vi "2020_day02.vi"() -> ()   [LabVIEW 2021]
panel:
  in  "Live/Test Data Src":bool
  out "Number of Valid Passwords (Task 2)":i16
  out "Number of Valid Passwords (Task 1)":i16
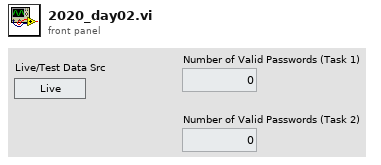
[diagram p1: front panel]
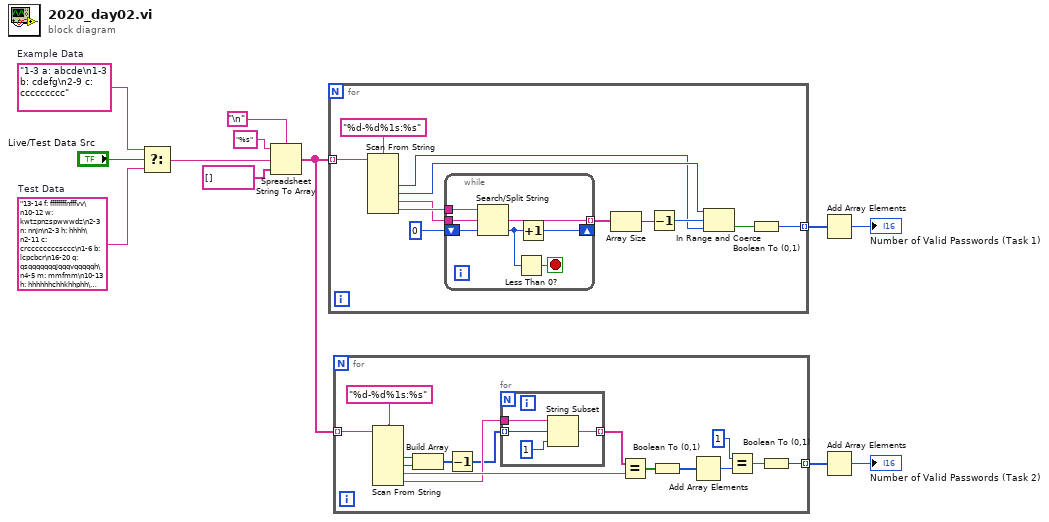
[diagram p0: block diagram]
diagram:
  w2 = "13-14 f: ffffffffnfffvv\n10-12 w: kwtzpnzspwwwdz\n2-3 n: nnjn\n2-3 h: hhhh\n2-11 c: crccccccccsccc\n1-6 b: lcpcbcr\n16-20 q: qsqqqqqqqjqqqvqqqqqh\n4-5 m: mmfmm\n10-13 h: hhhhhhchhkhhphh\n10-14 x: xxvxxxxxxvxxxwx\n2-7 v: tvvgvrvvv\n8-11 j: jjjjrjwljjzjkmc\n2-5 t: xtpftb\n4-6 m: mmmlmpm\n9-14 h: hhhhhhhhhhhhhchh\n10-11 x: xxxxxxxxxxx\n14-15 z: zzzzzzpzzzzzzzkz\n5-6 m: mwjmmw\n2-4 r: rrrr\n7-11 v: vvkwlmvkvkmbwvvvv\n16-17 j: jjjjjjjjjjjjjjjhj\n6-12 v: vjvvddtdpvvvldvqvdhv\n3-16 z: rktsvbkctznjkjzz\n5-6 r: hrrrrr\n1-3 d: ddxddd\n19-20 s: sssssjssssssssssssss\n17-20 b: bbbbbbbbbbbbbbbbbbbb\n2-4 m: mslm\n2-5 b: bbbbbl\n3-4 j: ljjj\n2-4 h: nlhbh\n4-5 z: zsmwfz\n4-5 j: jjzqj\n9-10 r: rrrrrrrrrj\n7-18 l: lljlgpmlltlzjltplln\n1-6 l: zbmljsljdszwl\n3-6 h: hhfhhqhhh\n10-14 d: vmddcdhsdzkxdddddddd\n6-7 s: psssssms\n1-10 j: cndjjjjjjjjjjj\n4-14 x: xxxdxxxxxxxxxxc\n6-7 f: fwfffsff\n2-11 v: dmmvlvsvvbbr\n7-8 l: dlcllllllll\n4-5 m: mmmmc\n4-10 m: zmmmlmnmrj\n5-6 s: ssshdsvbsk\n1-3 p: pppfps\n5-6 t: tttttt\n6-15 z: zzzzzzzzzzzzzzzzz\n7-12 m: bgshdmmkmmmmmfnmmm\n10-11 l: gclgllsllll\n3-4 d: dpdd\n2-9 n: kgngnrcxd\n8-10 n: knnsqnnnnrn\n8-18 f: qhwqbwnfppkffwhjjxf\n2-4 j: zwksc\n3-11 s: nkszjxwhcms\n8-11 b: tbbbbbbwbmbjk\n7-8 z: kvxfrzzzz\n2-5 g: hhwgv\n1-5 s: lmkxjbbsmnq\n2-7 p: spgxbpp\n2-8 z: xqzpztbvk\n4-7 r: wrtcfqrqcrlr\n2-4 g: gzgggg\n13-15 q: qqqqnrqqqbgqnqt\n7-12 h: dhxhbcqhhhhd\n7-8 l: llllflll\n5-6 d: ddbdfddwmndc\n3-10 j: jjjjjjcjjjj\n16-17 x: jhmqjpbpxsttjpcxrz\n7-14 j: jqjjjgjhjjmjjfjj\n5-7 l: zllllll\n9-13 d: dddddddxrdcsjdngbtd\n13-14 k: kdwkhqkkkkkknkk\n5-12 c: zcxwcbwfclccm\n14-16 x: xxfxxxhxxxxmdxxxxx\n10-11 x: xxxvxxxxxqxxxxxhx\n6-11 d: ddddddddddtddd\n1-3 j: bjbcj\n8-10 p: pppptppzpp\n3-7 z: zwldzgvztmbwwqwb\n4-5 h: hhhrm\n4-7 v: vvrvjvsz\n2-4 w: prsdkgxw\n1-4 q: fqqvqqqnm\n5-6 k: kzjbpkkkzzktkc\n12-15 s: ssvssssnsssdssgss\n3-10 w: wwfcwcwwwrjww\n6-7 t: thftndnvtztztb\n1-6 w: qgzppbcdjbpwmsj\n3-16 c: nccccfccrrcqhwcjck\n7-10 b: bfscxbdbnb\n4-14 x: xxrxsgxxwxptxxxdxdx\n1-4 c: jccb\n16-17 p: ppkppppppppppppwk\n2-10 z: wqtzzbhzkv\n9-10 b: bcbbqwcbbdvbzbfbsj\n6-11 s: ssssswsssssg\n3-7 c: wdcxzgtcrswqj\n4-10 c: xszcrmcsxccbwccxwv\n6-9 f: pffffffff\n7-8 k: wkhkhdkkkkkkrbkk\n3-4 q: cqqbqpg\n3-15 s: sswvssssswssssh\n19-20 k: kkkkkkkkkkkkkkdkkkkx\n11-14 d: dddddddddddddnd\n3-4 l: llll\n3-4 t: bvtvtrr\n13-16 b: bbbbbbbbbbbbbbbb\n16-20 b: bbbbbbbbbbbbbbbkbbbw\n10-11 v: vhvvvvvvvnvv\n1-6 v: xsvmvvxvkvv\n4-7 t: vttltqg\n16-20 b: bbbbgsjbxkbbbbbbrbqb\n15-17 c: ccccccchcccccxphcc\n1-3 w: cmwbtnzwwlhr\n2-16 j: njmqdfdsmrsptrjz\n12-13 r: rrrrcrrrrrrdhr\n11-14 j: jgjjjjjjjjtpjh\n4-5 w: wwstw\n5-6 w: mwrgwwmdwhzk\n4-7 b: bbdlbbbbc\n1-16 b: xbbhfbhbbbdbbdbbbbb\n11-14 h: hhjhjhhhhhhzhh\n2-3 t: jrtrt\n5-6 w: pdwwww\n5-16 m: mmhrmsvmxmvjdltm\n15-17 b: rbdbbbbtbfbbxbbbbbbb\n4-6 t: lzjtttqdpthkzrt\n3-4 x: xcxxxxxxxxxx\n15-16 z: zzzzzzzzzzzkzrcljz\n15-20 b: bbbbbpbbmbbbbbbbbbbb\n15-17 z: zzzzzzzzzzzzzcqnzzr\n3-13 t: tntttttttttttt\n6-10 s: jssmqsslsssddtg\n9-10 p: ppppppppjp\n9-14 d: sdxnfmpzlgvdcs\n5-6 c: cccscvcc\n2-4 r: rrrr\n11-14 v: vvcvvmvvvpvvvjv\n2-6 h: znfjphzqzdczp\n5-12 j: msdjjbjbgjjjbl\n4-7 h: hhhthkhhh\n5-6 q: qqqqqc\n18-20 q: pttqsnjcfchtfnqbjlqf\n11-12 x: xxxxxxxxxxxq\n5-6 j: xqbwjjcxjjljgj\n7-14 g: pdkdbzgzjvdvwggpnnt\n2-17 j: zhklmfrwspkgqbxjjdp\n5-17 b: bbbnbkbbbgbbxvzxhb\n6-8 b: bwhbbbbb\n6-16 q: lgxlqsqqwwmqrqqfgp\n16-20 j: jjjkjjjjjvjjjjjjwjjb\n1-2 g: vggg\n3-7 v: fvsvvxfvvv\n5-8 q: vdqqqqqqcrqqxq\n11-16 w: wwwwwwwwwwbwwwwnwww\n5-7 s: swwzsss\n3-6 d: hqwqcvdnqvh\n2-7 h: hsqhthghhhh\n4-9 d: dddtddddddd\n8-9 d: ddddddddd\n2-4 q: qqqsq\n4-6 t: ttnlqt\n4-6 s: sssszscs\n2-7 l: ssfllslplqll\n1-3 m: vmmlm\n6-13 q: qtqqqrqqqqqqqqqq\n2-10 d: zbldzlzssd\n4-5 n: nnndq\n8-18 b: wbbdgkvgscbdgqvxdj\n5-6 r: srrtrrrrr\n6-8 m: mmmmwbpm\n11-14 h: hhhhhhhthhhhhm\n2-4 p: pvpxpp\n5-6 g: ggvgng\n4-5 x: xxxtp\n3-10 v: vbvvzvhvvvvmvbcvvwrv\n11-13 d: ddddddddddxdldd\n4-5 g: gggggggggggngfggg\n7-8 j: jpjjjjhw\n2-6 m: jmfrmmhhsgbmmm\n6-10 v: vrvvvbvvvsv\n8-15 c: cctrcccpccccgcc\n14-16 d: ddddxdsdzwdddwdsddh\n5-6 m: mmnmmb\n2-6 d: dtwlswdnlkn\n12-13 x: vldxvmxcnndzx\n4-6 k: kkkxkm\n1-4 p: pppp\n11-16 b: bbbbbbbbbhdbxpbbbpb\n1-5 j: jjjjjj\n6-8 q: zqwdqszvqwqbrmhfqqm\n2-5 q: nqqczhb\n12-17 v: vvvvvvvvvvvtvvvvpv\n1-3 w: wwlww\n9-11 n: nbndcjnzntnvjnk\n3-4 q: qqcr\n15-17 p: plppppppppbppppplpp\n1-2 c: cvdlsccrccldccvfcc\n4-5 p: bpppcp\n19-20 d: dddddddddsdddddddddd\n2-4 t: bwbtmjbgkdlpjkrxt\n2-5 l: llxdblrcvnpclt\n11-13 b: bpbbbbbmbbbpbtcbbbzm\n6-7 p: ppppppp\n5-18 m: mqmmqpmmmmmwmpmzchms\n3-6 g: ggggmggkgg\n11-18 z: wjwlzzptzzzwbmzzgz\n5-7 b: bbcxbfbwbbcn\n4-5 p: szppp\n2-12 b: bbbbbbbbbbbmbb\n6-10 m: jmmmmwmtmfcwwxm\n4-5 m: mrqzmmmptfkmch\n13-15 q: qqqqqqlqqqqqqqqd\n1-5 b: kbbbnb\n4-5 t: qdtttszwwppbtllp\n12-14 c: cccccccccccccm\n4-5 g: gggdhg\n1-4 b: wbtbb\n3-6 d: ddrdgbdvdv\n14-15 x: xxxxxxxgxxxxxvdx\n13-18 l: lllllllllllllllllll\n5-7 p: zjsxppv\n4-13 v: vvvpvvvvvvvvf\n17-19 q: qqqqqpcqpqqgqqqqqqmq\n1-5 r: rlmrrr\n8-9 j: jjjjjjjjw\n2-4 q: dswq\n16-17 z: zzzzzzzzzzzzzzzzzz\n4-7 h: hhhzhhw\n11-12 l: lllllhhpllllqlllln\n11-12 h: hhhhdhhhhhrhh\n3-4 j: pkthmjsjqx\n15-18 b: bbbbbgbbbbbbbbbbbh\n4-5 j: lsxklmdwmhj\n1-2 p: pptp\n8-10 g: fgggzrnggg\n3-7 k: njkdhpkpqtqxhqwkp\n10-11 l: llllllllllz\n12-14 q: qjqhkqmqqwqgqcg\n1-3 m: mmmm\n8-19 c: dwzvhvbcpdbhcnrlcncx\n3-7 x: xtxjljw\n6-18 t: pttgnchttttttttqtt\n3-4 p: pppxpp\n15-16 k: kkkkkkkkkkkkkkvr\n2-3 x: dxxmx\n12-20 m: mmmmmjmmcmdmmmmmcmmm\n6-13 h: sthvjhlhfhxlhb\n4-5 t: pbrlttgmmwztxtrt\n3-7 p: dpptmppp\n7-9 p: hpppppppp\n3-4 q: qdgqqq\n1-4 c: cffcrkpdczhbj\n1-8 d: cqdwddlrddd\n9-10 n: gnkmnxnzmn\n3-4 k: kkxx\n1-7 d: vnddddn\n8-12 l: jllnlcllllllllvllb\n1-4 n: nnnnnhnnnn\n9-12 s: tssssszsssssbt\n8-13 h: nhnhdtkjbsfvbsh\n2-4 v: qmvs\n3-6 c: chcxccch\n1-5 d: ddddd\n11-15 l: pklllvllwlmlcklllll\n1-3 v: dvkbwsgjzqzzjmznd\n5-6 j: zjjjjjs\n1-4 f: vbffrwfr\n3-5 x: xxxxxrfdxmnbkrjbdzcx\n16-19 s: spsssbmrpbwrhqssgft\n13-15 v: vvvrvvvvbvvvvvv\n6-9 q: lqfqgcwtdqzgrqqp\n3-5 w: fwpwx\n7-8 h: hnhschhfphjzphwh\n2-6 r: rrrrrrr\n8-10 h: hhrhzhhttm\n9-16 w: wwwwwwwwfwwwwwwh\n2-3 n: zbnfnlpcnjqftpv\n14-17 k: rqwlkzqczczrlktcl\n6-7 f: ffffffff\n3-6 k: nndkjtpjzpmkkr\n12-17 p: gpppbpmjpptpfnzpb\n16-17 n: nnnpnnlnnnnnnmnnnnnn\n4-6 r: rrsrwr\n4-7 x: cnljrzcj\n7-8 s: srgtqlmc\n8-10 n: nnnnnnnvnn\n2-5 g: ggqggb\n7-8 h: hhqhgpxb\n4-12 b: bxbchbbbbbbbb\n2-4 z: qfzng\n6-13 m: pcmmwdkmzlstn\n3-4 v: qvdc\n2-10 t: tktttttttmt\n9-15 t: tttttttttttpttw\n8-13 p: pppjpppkppdlv\n6-9 g: gggggngqg\n2-9 k: lzvkqkkkkk\n8-12 h: ldpnjvchhshx\n5-14 c: cccccvrccccdbccchjc\n14-19 k: kkjksgrrkklhkkkkkkt\n5-15 r: hrrrrrwmrlrgrlz\n7-17 g: hbjtgsxbgrgggcjlk\n4-6 q: lqcbqvzqrqzqxqnqd\n5-8 x: xkdxsxxf\n12-16 m: vxlfjgzgqhxmlvmmqmm\n2-13 c: vccvjvqrgrsrqv\n4-6 l: ltlrlpvnl\n12-16 p: ppptdppppppcfppzpgsm\n18-19 q: qfqpvwpwjqvlnrmvsqq\n5-6 m: mmmmmh\n6-7 m: mmmmsls\n3-4 p: pvcg\n6-7 h: hhhhhhj\n1-4 g: gkggc\n3-10 n: sqsndtgnjbnljnn\n5-11 h: tcmlhlnbfnhgt\n9-10 t: ttttttttxl\n6-8 x: mxvxxxxhxxccbx\n9-16 g: rgggthgxggdggjgg\n7-20 w: wwnwwhvmtwnvwwpzdxvt\n13-14 t: tttmttlttgttlptt\n5-6 f: ffffpg\n5-7 z: qzzzzzqzz\n1-3 b: bfbfdhkwdzttcldtr\n5-8 n: nnnnrnnqnnnn\n7-18 m: hgnrbdmvmzqmhnhhpww\n2-6 h: rjghpwxhn\n5-10 m: bjqjmmnbvmlxpvvdds\n3-4 v: hvjttv\n4-8 n: nnpnnnnnn\n1-10 g: gzxghcgkggggtxg\n4-6 b: pbgblbbb\n4-7 c: ccccccmc\n2-4 g: ggwgtzvxqhjqphfg\n3-5 t: htdtt\n8-9 t: tttttptttttt\n4-5 v: dvvvd\n6-12 p: skzhnpblmpppcptfpll\n15-16 l: llllllllllllllvp\n6-11 b: mbbbbjxbbmbbf\n2-4 t: mtqwtnt\n2-4 h: wfhkh\n5-6 w: wwwlwwwkw\n7-8 k: kskkkktz\n5-6 g: rggqcv\n2-4 z: krmw\n2-4 q: qqwqlrqcbxlxbpqg\n14-18 m: mmzmmmmnmmmmmtmmmm\n1-5 p: pqwfpnp\n3-7 w: dwwxdwgwwksm\n8-11 g: bkmcfcddjvw\n7-9 s: srsszspss\n3-4 r: rjrsz\n12-14 k: kkkkkkkkkkkgkl\n13-14 f: fffffffffffffh\n7-9 r: qgxpglrlr\n4-6 l: xflkll\n2-9 d: gdddddddrqdddd\n2-3 k: zskkzq\n3-4 z: jzrtwgmtl\n3-4 b: bnnbbx\n1-9 r: rhmrwwrfmsb\n7-10 b: btbbbbbbjbbb\n7-8 t: lmttpttq\n1-4 s: rcls\n11-12 k: kkkkklkkkskq\n14-15 p: ppppppppppppppp\n3-7 l: dcslvkjgjcdk\n1-6 l: hllhllpl\n6-9 z: zdlqztzzkzz\n10-11 r: rrfrrrrrrrqjpkkrmrrh\n4-5 v: bvpqvvkvrxnvzmghbhmx\n10-11 v: vvvvvjvvfcvvcvpj\n10-11 j: jjjsfhdmjtcvbzj\n4-5 z: zzzzzz\n14-15 l: lllllllllzlllkcnl\n3-8 c: dchcjjrccvm\n12-14 b: vrwbfbqbbbbkbhgqjjh\n8-9 g: stggqgctgpgggctt\n15-17 p: pppppppppppkppqpp\n7-8 q: qqqjvqhmqq\n3-4 x: xxxxx\n7-8 g: ffbgglgzpjgqvnglpsgh\n14-16 r: rrdrrrrrrrrrrgrrrd\n10-13 l: lllllllllllll\n6-14 q: qfqzqnqqmhqqsp\n2-3 q: qqqqq\n17-18 f: ffffffqfffffffffftf\n11-13 h: hhhhhhhhhhmhz\n3-10 c: cccmcccccfzc\n8-12 v: vvvvvvvvvvvvrfwrvv\n3-4 v: vrnx\n1-12 v: gfvsvkvvvzvcvsv\n9-10 b: lbtgbbpcfbgb\n6-8 f: fgnffkfshhfbfc\n8-10 w: wwwwwwwwgpltzwzk\n7-12 b: btbbjbhbbpbbqsbbbvp\n11-12 r: vfcvrrrzrhvc\n19-20 g: gggggggggggggbggggjh\n11-14 s: sfsvsfsswsssscxssm\n4-6 c: lcclcc\n7-8 g: gggggggr\n10-14 g: gdcpmgxlgggggtgbgg\n2-3 b: bktb\n9-13 k: krkkkgkkkkvkkk\n2-12 f: bwtgngzflzcfchx\n2-4 m: mmmmmmm\n10-12 b: bbbbbbbxbbblcbpb\n3-4 c: ccct\n6-8 r: kgqvrrrjn\n10-12 f: ffffffwfffff\n6-7 c: ckcjcjccc\n10-12 l: lllltllllllxll\n3-6 q: qqgqqlxqqq\n4-5 b: nbbbbb\n7-11 r: rrrrrrrrrrrrrrr\n10-11 s: sssssssssss\n1-6 w: wwwwwwwlww\n5-7 l: lrlmlll\n8-12 c: fbcmjxccqcwc\n9-10 b: ljmbxwbbbbbhbbb\n2-4 h: shwgvlw\n15-17 t: ttptttttktttkttttt\n2-5 d: dddgdd\n2-14 x: xbbtnzdvbszrlxl\n8-10 c: cccccccbcx\n10-12 k: kkkkkkkkmkkc\n7-17 r: rzbcshqhmrzrktzdr\n5-16 k: kvkkdkkkkkkkkkklk\n1-7 p: hkplfbjdhsh\n1-6 z: pnzzzz\n12-18 m: mmmjmxmmmmmmmmmmcd\n5-7 k: kskkdbsk\n9-10 b: bbbbgbbbbw\n4-6 c: cccccjs\n19-20 w: wwwwwwwwwwwwwwwwwwwf\n7-11 j: drzjhxkjjjkwr\n10-15 c: cccfckccccdccxc\n1-3 d: ddddc\n13-14 j: jbjjknjjjjjjjjjjjzzc\n1-4 m: mzmftx\n1-4 t: rttt\n12-17 t: tltqttzttttjwcttrwtt\n6-10 m: rmfmrnmmmdmqp\n6-15 p: jpfpppwppppppznpppp\n4-8 p: mppxctpb\n2-4 z: gwzzrn\n3-4 p: ppfpp\n3-4 b: bbbh\n11-17 l: llllllllllllllllhll\n4-6 m: mmmmmmm\n4-6 c: ccccjx\n11-14 g: gggggggggggggg\n3-4 l: llflq\n9-13 p: pspvvcpkpcpzpfpk\n1-4 n: nhwn\n6-10 j: jjjjjjjjmjj\n9-12 p: ppgpwxpplgppzpppwpp\n10-14 h: hhhhhhfhhhhhmxh\n8-10 l: llllllmcwfl\n7-8 h: hhjhhhps\n8-11 v: grvvvgbvxvvlhvvbdvr\n5-6 m: fmjjbmp\n1-2 x: xxhd\n11-15 n: nnnnnnnnnncnnnm\n1-8 g: jgggbggd\n13-15 l: lshllllllllllll\n5-12 r: crrsrrrrprtrr\n10-16 k: hkkkkkkjkgtkkkkkq\n5-16 j: prxjxjjdxzjjvjjwfj\n7-8 k: pdkkkkkzkzw\n3-4 s: sstg\n1-5 x: vxxxb\n10-16 s: tqmzsfksjzfmlqzsdb\n2-5 r: rcrxjr\n10-15 v: jcbvvvhvvvkwrgvvvvv\n4-6 n: nnxnnpnn\n13-18 l: llllllllllllbllllgl\n9-11 g: vwqgnrzlclgqtp\n2-3 f: fpms\n3-5 l: llllllll\n7-12 x: xcvxzxxhxxxxxxxxqxxv\n6-10 b: fcfpwbmbhbpbbqkkbxb\n8-11 z: nrnzzqzzzzck\n8-9 g: nggdfgdgggfggg\n2-6 d: sdztkkfvpkddggdxd\n10-14 g: nhdstmlfxcggcs\n10-11 g: ggzfglgggmcxgjh\n3-13 x: cxjxxxxxxgxvj\n9-10 h: smlxphtmkhf\n7-8 v: rhdvgcvrdvvvvvxwvssh\n7-14 n: nnnnnnncnnnvnn\n3-6 z: zzzgznzz\n6-10 l: llwmgllljllll\n4-5 v: vwvvpvw\n7-8 m: mmmmqvmqmv\n13-14 z: zzzzzzzzzzhzrcz\n3-8 h: bdmhcxpgbpjvwfmh\n3-5 h: nhhjk\n11-19 b: zrrmrqbfvwbnmvkvbzbv\n3-8 c: ztwqhccmwzvcbxjjrc\n4-9 h: hhhhhhhhh\n2-15 d: lddzlxhkscrmfbd\n3-9 s: kpscwnwzj\n10-11 w: zwwlwxwwwwwwww\n4-5 v: dpvjr\n1-3 d: ddtd\n3-6 x: xxdfxxxrbdh\n3-6 g: dghwgxg\n8-10 z: zzzzzzzpzz\n13-15 p: pjpxpppppdcpphlppjp\n6-16 j: jjjjjljnjjjjjqjjjwx\n11-17 f: fffffffffflfpfffxff\n8-10 j: jjjjjjlwjkjrdjjjj\n8-9 w: wwwwfwwdkww\n4-9 x: qpxbhxwxxkx\n5-7 w: wwwwbwl\n1-6 m: mmfrmmmm\n8-9 l: lllllvlsl\n3-4 d: dddd\n6-8 c: cqcptcfcgcrzbjcccp\n10-11 k: dccpkmkkgkkdzkkkkkk\n3-4 j: jjjr\n3-9 h: hzhwhchzhjg\n7-8 g: bxgnvvzfsbggdgg\n2-17 f: ffffffffffffffffffff\n7-13 g: ljggdgztggvgtggg\n9-13 x: rxlxrxxnwqxpcdxq\n10-11 j: jjctjjjjjfjj\n8-16 k: zpzskgkkkvsbxhsk\n4-5 l: llljl\n2-6 b: bbbbbb\n1-3 w: swww\n6-8 r: rrrrrbrbrr\n8-9 t: tttttttth\n3-5 s: sssss\n3-14 q: qqxqqqqbblqqcqmqsq\n7-8 v: dmfvccvvvbvmwjvvvqfv\n5-7 v: qvvvvvvvv\n4-9 c: cgcgvncctwrtv\n3-5 p: ppnpppp\n13-15 h: hhhhhhhhhhhhhhhhnhhh\n5-8 r: rrrvpgrdbhrc\n2-9 q: szlqwzwhqxbxkr\n5-6 c: cwrmhxcpxchzccb\n4-6 z: zzjczz\n12-14 p: pwqkbphzplxhnpm\n8-13 t: tkkzjttrstbtwttd\n15-16 m: mmpqmxbxdzmqmmmb\n4-6 c: ctcpczdd\n2-3 j: fdjjj\n15-19 k: kkkkkkkkkkkkkkpkkkwk\n2-3 c: cccc\n1-2 w: wwfqwwgpmv\n2-3 h: wfzmhm\n3-10 s: wbsbvhfxjgxfqstwqn\n15-16 r: sxrzvkqpqmgzgtrr\n3-5 m: fmmtmqjxzss\n12-13 k: ddsnpkfvknhwq\n5-11 z: lzwvzhtzzzz\n12-13 t: tttttttttbdgtft\n14-19 g: gggggggggggggggglgnv\n3-4 r: rrrr\n3-7 h: xchhnhh\n10-11 n: ndnjnnhnnnk\n5-7 l: llllhll\n3-5 p: ppppb\n11-12 s: rrsjzvswsdtxssv\n2-10 z: ztxzzzzzztzp\n16-17 m: mmmpmmmmmmmmmmmmmmq\n1-6 b: wkbfntzw\n10-14 n: nnnngrnnnnnnnnnn\n1-3 b: pbdfsbbp\n6-13 n: brnwnhnnsnnrwncnmz\n2-11 f: mlhpdjflklzmhxt\n1-2 f: shzsffl\n8-16 k: kkkkkfkxfwnslkkm\n13-14 b: bbbbbbbbbbkbqbb\n2-7 x: zdxxxxxx\n6-10 h: hhthmpvhnlk\n6-7 p: tppfpqpcppppxpmpcpp\n3-5 m: grmkm\n5-11 w: vcwbwwwbwwswnrdwfwx\n1-6 s: sssrssssx\n13-14 j: jjjjjjjjjjjjgj\n14-19 q: sbqqzqnqnlzdrlqqqtkl\n3-4 t: btdttvzrvnjst\n1-7 s: ssbsssmhssssdsc\n3-4 z: vcdzj\n6-13 v: vvvvvvvvvvvvvv\n2-7 t: ttttgpthqhmth\n5-9 z: zzzzwzzzl\n10-15 w: wwwwckbzwwwwkwwlrwb\n2-7 r: wjrbdzrjxrstrc\n1-8 z: dpzzzvcsx\n4-6 c: nccxccvcccczcccdc\n1-10 c: cccccccccc\n3-7 d: zdmdpdntdpzncdbff\n5-9 x: xvlvxldrxxmbdcdxxxz\n6-7 p: ppplppjcwcpp\n2-7 d: pwnhpdd\n2-3 q: hqqsdqxs\n6-9 t: smttzjmktq\n7-9 t: ttttttttp\n4-19 w: wwwrwwwwwwwkwwwwwwnw\n17-20 s: cssvssssssssssssssss\n10-11 s: srssssssssss\n5-6 f: ffcfjt\n3-4 d: ddgdddddddd\n2-15 s: sssssssssssstsssssss\n2-4 c: kmccnnt\n2-3 f: ffff\n10-14 s: vspjssnsssssshvsq\n9-10 k: skkkkkkfxkkwk\n3-5 g: mgnggjpgspcf\n4-15 z: zzzdzzzzzzzzzzzz\n3-4 c: cgcc\n6-7 s: sssssjs\n2-4 z: ztzz\n17-18 w: wbqwwnwwwmwvwwhgdnl\n13-15 d: dwddddddddddwdddd\n4-7 g: gzghgcnq\n3-9 n: snnnnnmll\n2-7 j: sjhtsxj\n2-6 h: khvzdhhr\n2-10 t: tttttttttttttttt\n4-6 x: xxglxwjrx\n3-4 r: rjrc\n5-13 b: bbbbbbbdbbbbbb\n3-4 q: qqrhqq\n8-12 g: ggggkggdgggbg\n3-12 j: jjjjjjjjjjjjjj\n1-5 c: cbcch\n10-11 r: rrnrvrrrrzn\n4-16 j: jjjpjjjjhjjjjjrjjjv\n8-9 f: fffffzdsvfccfr\n14-16 f: ffzfjfftfffffffffff\n2-8 n: ngnnnnntnnnnr\n6-11 n: nchnnvnnnndn\n4-5 w: sfwvm\n6-14 s: ssssssvsspssqhsss\n3-4 m: sjjb\n2-4 d: dnkjd\n3-9 s: twsgkmqstq\n6-14 f: ffffffffffhfff\n10-15 w: wmwlwwwwfgwwjrzwwwww\n3-11 f: fffffkxfffffmfff\n1-2 l: jlrpl\n3-14 p: pbnpkbppxhppmpp\n1-14 v: bvvvtvvvvbvvvh\n3-4 s: zssvs\n3-4 l: llljrlk\n8-12 f: ffcfffczlffff\n3-13 m: xsmgpvzsrrwmxtbktsrj\n5-7 j: qxvjjlqjjjjj\n3-4 r: rbdwg\n13-14 d: dddddddddddddg\n10-12 f: lqvhjnkfrfffv\n6-7 n: njnnnhz\n11-13 v: vvvvvvvvvvvvs\n12-13 v: nvvsfvvvvvnvdvjxvvv\n2-19 s: slsssssbsskspssssts\n9-11 n: nnnnnnnnnnm\n4-5 j: mhngjjrhjcjkjw\n12-18 p: pnfwppppprsqrppltppp\n9-13 s: wsssfsjsssfssss\n6-8 b: bbbbbzbj\n9-12 c: lcccccrccctv\n7-11 w: wbdwwqwwkbwws\n6-19 c: cccrmldccfhtvclcccc\n9-14 h: bhhhhdhjkhhhhm\n7-15 g: gkgggggvcgggghgggz\n4-8 k: kknklwkkkg\n10-13 c: ccccccxcccccccc\n10-14 c: ccbcfcccptcczbcc\n8-9 s: scsssssss\n1-7 v: bvvvvvvvk\n4-8 s: dspsskkstklsz\n9-10 b: blbkkzbvvpbhbbbb\n1-2 m: qgntnbccqm\n7-14 w: wwwwlftgspwmwr\n4-13 n: tnxmnnwwnnlnnnnz\n3-5 c: cwzbs\n3-6 d: dddddl\n6-8 s: qsfssrnsst\n1-2 l: llxcx\n9-11 g: zhzkcbglvgw\n5-11 f: lfzgtbcmzzw\n6-19 m: gcbgjbqrdkswqhmxjct\n1-3 z: dzzz\n9-13 t: wttftcddttmtttgttnvt\n14-15 z: zzzzgtzzwzzzzzzzzz\n1-11 q: qqqqqqqqqqqq\n4-5 j: rxjjjxjwjjj\n3-5 v: gqjhjvlvlbmkgssd\n16-17 q: qgcbftwncjhdzwqmw\n1-3 g: tjftgp\n11-16 l: rlllllllllgglllm\n4-6 z: zprzvrfbpblf\n7-11 j: jjjjjjjjhpjmjj\n3-4 l: ltlrblllwljljlc\n8-11 k: kkvkkkkkbqkskrkkd\n5-10 r: hjrcrrrdvtrkrvrxrr\n5-6 x: xxxxpx\n13-16 g: gmggggggcggpwgghgt\n3-4 h: hzzp\n13-15 h: hhwhhghhhhhhhhh\n3-5 t: mlftttt\n8-13 c: cccccvcdccccfcccccc\n1-6 k: kczzpq\n8-14 t: rtcttttgtttttgtttz\n6-7 l: lhsvlll\n1-2 x: cxlr\n8-10 t: rtbtttttsblttttb\n11-14 z: zzzzzzzzzzdzzzz\n2-3 t: ltttbthjdxwbxrv\n5-6 x: xxxxxxxkx\n8-12 f: fffffpffwfng\n5-6 x: xxxxflxxxxx\n5-7 d: ddddvvk\n4-8 j: ttjjjjhj\n2-5 p: rtrmpksjdvpplmrkl\n9-11 s: ssshsskssssssr\n5-8 j: wjnjjvjjfjjhf\n4-6 q: qlpcjqqqq\n13-14 m: zctdnmkjstxbmmfqtns\n4-11 n: nqntnngnvmnknrnwnnl\n3-5 d: ddfvdnkd\n9-14 j: wsznlrpljmjwjjjkmtk\n2-6 w: wlwwwww\n9-12 j: jjzjxjjjjhjp\n10-13 v: zvvvvvvvvfvwlvvvv\n3-18 x: dzxcqgwxpwxvpmcxxdxx\n2-3 w: wsgwwd\n3-20 n: nrnfxnnnnlnnnnnfnrhp\n3-8 f: fmvjwsffvxjfnlw\n5-6 l: llllcs\n3-5 b: bbbbbbc\n2-7 l: rlwkflnsm\n4-18 m: dqskhdqgmrpbgtmdnp\n4-6 r: grpxzr\n5-7 m: mmmmmmjmm\n7-8 b: bbkkbbkbb\n1-4 r: rwrtr\n5-6 g: gggcggg\n4-6 l: qlcbwrsf\n16-18 t: tttmtttltvtttttxtrtt\n3-4 z: zzzz\n6-10 g: gggggtgggg\n12-15 f: tffffffffqrffvvftffh\n10-16 w: wwgwwpwhqdwhwpbw\n5-7 m: mpmmmmm\n3-5 b: bbxtbbb\n5-10 x: xxxxbxxxkjkx\n10-12 b: bjbldbbbwbxg\n3-4 g: gnggqgg\n2-4 s: sstst\n6-10 j: jjjjfvjjjj\n16-20 r: rrrrrrrrrrrrrrrrrrrr\n4-12 b: bbbxbbbbbbbbbbbbb\n3-4 k: kkpk\n4-7 s: ssssqsh\n10-13 b: vbzbbbbnblbbb\n12-14 f: rgqffrfsvftwff\n2-4 x: bfxvhmsxnqxz\n10-12 c: ccccccccccbcc\n1-4 l: llxbmjpll\n9-14 f: ffhfmpfffffzfgcg\n3-4 n: ndfm\n1-6 k: lkmdzgfbkfktkkvkw\n12-13 q: qtkqqgqbqtqgvqqqzq\n7-9 d: ddddddhddsd\n4-11 j: kdqjjjjjjxg\n4-6 k: kkkgkm\n6-12 n: nnnnndtnnnnnnv\n2-6 c: dccccdc\n10-11 v: vvvlvvvvvvb\n7-10 w: wwwwwcwtzwkpvjqwsb\n1-5 x: xxxxxxx\n5-8 g: dhggzggsggggglgggg\n8-9 t: dttttttdtfnt\n11-17 g: cqgglgtwgggcbwjvwg\n1-2 t: ttttt\n16-17 j: jjjjjjjjjjjjjjjjjj\n4-7 k: lkdkhkkkfk\n15-17 z: zzzzszzzzzzzzzwzlz\n3-13 w: wwswwwwwwwwwfwww\n5-12 h: mstzhsghhhhnzmdrh\n10-12 h: hhhhhhfhhphhbhhk\n3-4 j: jjsd\n11-12 k: kkkkkkmkkmfd\n19-20 d: ddddhdddddddddddddxj\n7-8 g: gggjggrg\n4-5 m: mdzmv\n3-4 w: wwww\n7-8 b: bdbwbbbbb\n2-12 q: dxqqqqqjqqqlqq\n3-6 w: wwwwxwh\n9-11 s: smhnkssssssstxj\n5-6 n: nnpnkj\n7-8 s: qsgdxkjs\n9-14 m: mmmmmmmmsmmmmv\n1-3 v: vvcvv\n2-5 x: kzxgjttwxspclfx\n5-8 c: ccctpcckz\n5-6 h: hhhchthqxchh\n3-7 t: hnrcqdtttmtxtnmhcf\n2-4 v: vvlz\n4-5 k: kbgkl\n9-12 x: mhzpjqtxqnfrcnwhk\n7-11 z: slztclzvxbzmz\n13-14 l: ldllllllllllkcl\n1-2 l: fslcthfv\n12-16 b: bxbkbbbbbbbbbbbb\n1-4 r: rrmr\n8-11 d: dddfdpdddtdd\n17-20 n: nnnsngnbnnnnnnnncnnn\n1-16 x: xxxxxxxxxxxxxxxxx\n2-4 z: zqzv\n1-4 m: fnwm\n2-3 j: jqvd\n10-12 h: ghhhhhjhhchg\n14-15 v: vvtvvvvvvvvvvvv\n4-6 f: ffffff\n8-20 g: tgghjfglrzggggcxhcgg\n9-11 p: pvpmzppppkpk\n5-18 x: xxxxnxxxxxxxxxxxwlzx\n10-11 m: mgdmrfchqwmfmrlnq\n7-8 g: gggggzxs\n4-6 n: vjnchzknzbvnvn\n17-18 p: pppppppppppkppppjp\n6-8 d: dddddfddld\n1-4 r: brrr\n2-10 m: mzmmhqmmmmkmmwm\n8-15 f: cfjwxkgmfkxdmwxf\n3-8 c: djskjzcmwjcz\n2-3 k: hkckkjbztrggrffvxwm\n11-13 d: krddnddddrddgdddd\n4-5 f: zjsndf\n4-5 r: rrrgl\n1-2 z: tsbn\n1-11 s: sssdwtjssssskkszms\n6-16 x: xfxxtxxxxxxdxzxmxx\n5-13 m: mmmmmmmmmmmmmvm\n2-4 z: zdzj\n3-4 d: dddd\n3-4 n: nnmnkv\n14-16 d: dfddddddddddtddddqdd\n5-7 n: jnnnnnnj\n8-16 q: qqltjqqqqqqqsqqfq\n10-14 s: sssxsmsssvqjssss\n6-7 w: wwwwjwwxwd\n2-5 m: mzqcndqmnmmgwmsspm\n9-10 k: tkkkkrkkkhkk\n3-5 r: rxrrrrr\n7-11 c: glfcdqrcnfhc\n8-9 r: rrrrrrrjd\n7-8 d: ddddddlk\n2-7 j: pjsmjjr\n2-4 x: txxx\n13-15 f: ddkhqfnbcmtwvbf\n7-11 n: nnnnnnnnnnvn\n7-9 m: jmmmlgmmthlrm\n8-13 w: wwwwkwwgwwwwfrwww\n2-6 d: drdrhn\n8-10 k: lnkfrvgkzkchq\n4-7 z: lxjzzzzhzprrzzzpcwj\n1-2 s: lssc\n2-3 n: jmkcngpn\n3-9 x: xxmzxnxxxx\n3-12 v: nqwshwqgfnwvwvnf\n5-8 m: zmmmmmmmqlkprv\n1-5 q: qpqrqwqsvpjqf\n14-18 q: qqqqqqqtqqqcqqqqqq\n13-16 v: vvvvhvvvvvvvrvxdv\n2-6 r: rrlrrrk\n6-8 r: hmsrxsrkprdrrrl\n14-16 s: sssssslssgswssssss\n3-11 t: ctttvsnfcstzktktb\n1-11 c: gwfbddphwnqcmf\n3-18 h: hhhhhhwhhhhhhhhhhs\n7-9 c: cjjcrtpvctccfcc\n6-14 f: fffffgfffffffff\n8-15 z: zzzzzzzzzzzzzzdz\n9-16 d: ddddbdddhddddqpd\n1-2 q: qffc\n3-5 l: grcsjln\n12-13 q: qqqqqqqqqqqqq\n4-5 q: qqqlk\n1-3 w: wwwx\n3-4 w: kwwf\n5-15 m: pkwmgmmxspzxhmmrmp\n5-18 t: ttfthsbwntpcnttmwtc\n14-15 p: pjpjwppkpxpqkpf\n1-3 n: nnnn\n8-9 j: jjjjjjjbxj\n4-6 w: gfhwfwwmfx\n8-11 k: kkckkkknkkkk\n13-14 m: mmmmmmmmmmmmsqmmm\n2-4 s: tsrz\n9-13 j: tjvjqpnjjjlkwjjljrj\n3-4 f: xwfgf\n2-7 h: rhxshbh\n10-18 j: jjjjjjgbjjjjjjjjjjj\n5-14 n: fnwnnnsnnnncnpnn\n9-13 h: qhhlnhhhqhhhm\n3-17 h: hhfgzkhhjhrbhwdcpbnh\n2-4 c: qccrblqtcd\n13-16 s: ssjssqssssqsxssw\n10-15 n: nnnnnnnnnqnnnnf\n2-3 m: nmtl\n2-4 w: wqwdt\n4-7 v: vvvvvvvvvvv\n5-6 w: wbctwwwgj\n4-6 q: qqqttqzzwsxp\n2-7 r: rcrrrrrr\n10-12 d: sdmddcfdddzvdddddq\n1-15 f: ffffffffffffffffff\n3-7 r: rrwddcjgr\n2-11 t: tttttgttttttt\n3-6 n: nhxgnqnnfs\n1-3 t: pqtwt\n8-17 r: rrrrrrrrrrrrrrrrrrrr\n3-16 t: tktnpjtcthrhtqltq\n5-6 h: kcmkkqdrbhhxm\n3-4 l: llll\n1-14 g: gggdgrvjtqfgpk\n5-8 p: ppppplwcpp\n4-7 d: ddddtdmdd\n1-7 q: qqvxrqq\n8-10 v: pvvvgkqrvvgnvlvv\n17-19 g: sdgghgnggggggfbmggp\n6-8 x: rvjknxlx\n13-14 r: rrrrrrrrrrrrrb\n3-10 b: zbkmbbbbbb\n4-6 d: kdtbdmkd\n8-12 m: mmzmmmmmcxmmh\n7-8 n: gspnbfnp\n13-14 l: llllllllllllnf\n4-5 b: rzbbbxblvbwbrbbbx\n3-5 x: bxgrcxxrk\n2-4 j: jjjh\n11-13 r: rrrrrrrrrfrrrrrrr\n4-7 q: mwqqfqqqnwqwq\n2-3 g: sghvhggvv\n4-5 k: kkkkk\n11-12 s: ssssssskssgss\n16-17 g: dcgqnwtptvvlfkdgg\n4-5 v: vvvqc\n2-6 s: xsksrmrrd\n7-8 w: swwwwwfnww\n5-6 m: hmgchm\n6-8 m: mmmglzmmmhfnfqk\n2-5 c: bnjknt\n2-3 x: lxxj\n1-4 g: gqgpzgtj\n3-12 c: cngsrcvcjccxgcc\n2-11 z: zpzzzzzzzzzzz\n6-7 s: ctsxgslsjbstspgsl\n1-2 v: vnqs\n4-5 n: rnnwcnfl\n14-17 v: kvvvvvvvkvvvvbnvw\n5-6 h: hhhchhh\n1-7 d: vmcdddj\n14-16 n: snnnnnnnnnnmnnnhn\n11-16 h: hhhhhhvhdhrhhghn\n3-5 k: lckkknk\n1-12 t: tcttbpgtdwdxwddrxv\n1-13 x: jxxxxxxxxxxxfx\n11-12 l: llllflllllll\n11-14 p: qpphckzdppkjxz\n3-16 d: nfngxfjxwdpjvjcds\n4-5 b: xkbmb\n11-12 s: sssssssssshs\n15-17 t: tttttttttttwttttt\n14-15 x: xxxxxxxxxxxcxxgm\n3-5 t: wxlttc\n10-11 x: xxxxxxxxxtk\n9-12 h: hhhhhhhhdhhhh\n5-20 d: smdvdkdbqbnsdssfhdnd\n16-17 d: ddddddddddddddsvtddl\n6-11 v: kvvvvvvmvvdv\n2-5 r: nrrgr\n1-4 b: bbbc\n8-10 p: ppppptjpspkpppp\n7-10 w: pjhswvhdjqx\n11-13 c: cfcfccbcctgnccccvcc\n8-14 t: tttttttttgtttttts\n1-4 c: fcccc\n4-6 v: tvfvvvqvlkrpxkvvhztr\n3-6 v: vvdvvbv\n13-15 p: pwppppppppppppp\n1-2 v: pwbr\n15-18 r: xrrrbrrrgrpbrprrqrqr\n2-4 g: zgggp"  # Test Data
  w3 = "1-3 a: abcde\n1-3 b: cdefg\n2-9 c: ccccccccc"  # Example Data
  n1 = Select(t=w3, s="Live/Test Data Src", f=w2) -> (s? t:f=w4:string)
  n2 = Spreadsheet String To Array(delimiter (Tab)="\n", format string="%s", spreadsheet string=w4, array type (2D Dbl)=string[] []) -> (array=w5:string[])
  n3 = for {
    tunnel: w5 -> [w23] mode=indexing
    tunnel: [w13] -> w9 mode=indexing
    n4 = Scan From String(format string="%d-%d%1s:%s", input string=w23) -> (output 1=w15:i32, output 2=w16:i32, output 3=w21:string, output 4=w22:string)  [unwired: 6 in, 3 out]
    n5 = while {
      tunnel: w21 -> [w30]
      tunnel: [w29] -> w19 mode=indexing
      tunnel: w22 -> [w31]
      shift-right: [w27] -> _
      shift-left: 0 ("offset of match") -> [w28]
      stop <- w26 stop-if-true
      n6 = Search/Split String(string=w31, search string/char (-)=w30, offset (0)=w28) -> (match + rest of string=w29:string, offset of match=w25:i32)  [unwired: 1 out]
      n7 = Less Than 0?(x=w25) -> (x < 0?=w26:bool)
      n8 = Increment(x=w25) -> (x+1=w27:i32)
    }
    n9 = Array Size(array=w19) -> (size(s)=w18:i32)
    n10 = Decrement(x=w18) -> (x-1=w17:i32)
    n11 = In Range and Coerce(upper limit=w16, x=w17, lower limit=w15) -> (In Range?=w14:bool)  [unwired: 1 out]
    n12 = Boolean To (0,1)(Boolean=w14) -> (0, 1=w13:i16)
  }
  n13 = for {
    tunnel: w5 -> [w45] mode=indexing
    tunnel: [w33] -> w6 mode=indexing
    n14 = Scan From String(format string="%d-%d%1s:%s", input string=w45) -> (output 1=w44:i32, output 2=w41:i32, output 3=w43:string, output 4=w39:string)  [unwired: 6 in, 3 out]
    n15 = Build Array(w44, w41) -> (w42:i32[])
    n16 = Decrement(x=w42) -> (x-1=w38:i32[])
    n17 = for {
      tunnel: w38 -> [w49] mode=indexing
      tunnel: [w48] -> w40 mode=indexing
      tunnel: w39 -> [w47]
      n18 = String Subset(string=w47, offset (0)=w49, length (rest)=1 ("length (rest)")) -> (substring=w48:string)
    }
    n19 = Equal?(x=w40, y=w43) -> (x = y?=w37:bool[])
    n20 = Boolean To (0,1)(Boolean=w37) -> (0, 1=w36:i16[])
    n21 = Add Array Elements(numeric array=w36) -> (sum=w35:i16)
    n22 = Equal?(x=i16 1, y=w35) -> (x = y?=w34:bool)
    n23 = Boolean To (0,1)(Boolean=w34) -> (0, 1=w33:i16)
  }
  n24 = Add Array Elements(numeric array=w9) -> (sum=→"Number of Valid Passwords (Task 1)":i16)
  n25 = Add Array Elements(numeric array=w6) -> (sum=→"Number of Valid Passwords (Task 2)":i16)
